vi "Add Wall Class.vi"(8 "error in (no error)":errorcluster, 10 "WallRef":refnum<class "Wall.lvclass">, 11 "object in":refnum<class "Game Board.lvclass">) -> (0 "error out":errorcluster, 3 "object out":refnum<class "Game Board.lvclass">)   [LabVIEW 2017, in "Game Board.lvclass"]
uses:
  Game Board.lvclass
  Wall_class/Wall.lvclass
  Game Board.lvclass/Game Board.ctl
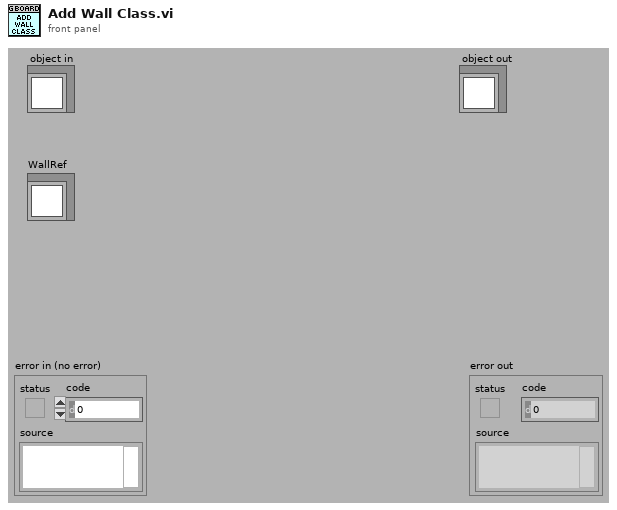
[diagram p1: front panel]
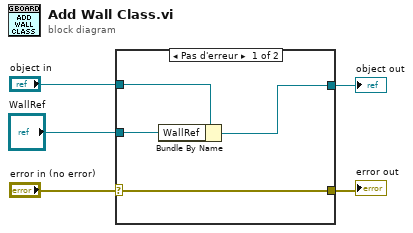
[diagram p0: block diagram]
diagram:
  n1 = case shown="Pas d'erreur" "error in (no error)" {
    selector: "error in (no error)" -> [w9 w11]
    tunnel: [w9 w11] -> w4
    tunnel: [w7 w10] -> w2
    tunnel: "object in" -> [w8 w10]
    tunnel: "WallRef" -> [w6 _]
    frame No Error {
      n2 = Bundle By Name(cluster=w8, "WallRef"=w6) -> (w7:refnum<class "Game Board.lvclass">)
    }
    frame Error {
    }
  }
  "error out" <- w4
  "object out" <- w2
